vi "deliverWater_RIG1_cue.vi"() -> ()   [LabVIEW 2017]
uses:
  <vilib>/DAQmx/write.llb/DAQmx Write (Digital 1D Bool NChan 1Samp 1Line).vi
  <vilib>/DAQmx/create/channels.llb/DAQmx Create Channel (DO-Digital Output).vi
  <vilib>/DAQmx/miscellaneous.llb/DAQmx Fill In Error Info.vi
panel:
  in  "element":tag="Dev1/port0/line0"
  in  "Water on time (ms)":i32=100
  # "RIG 1"
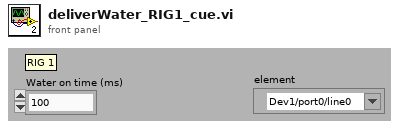
[diagram p1: front panel]
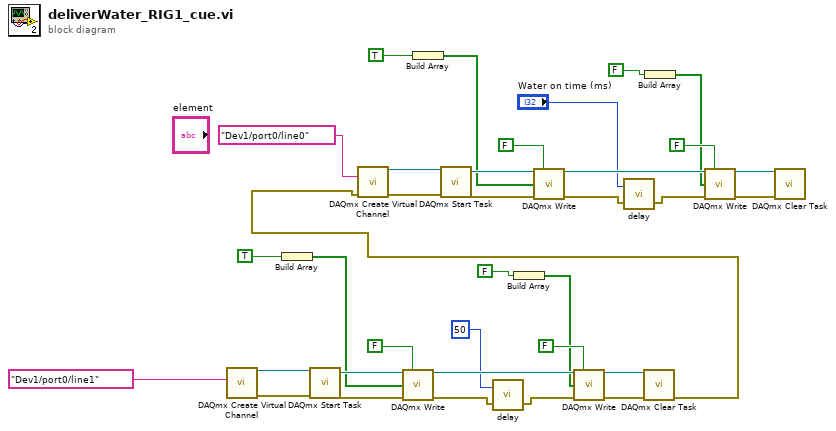
[diagram p0: block diagram]
diagram:
  n1 = call-poly <vilib>:"DAQmx Create Virtual Channel.vi"("lines"=tag "Dev1/port0/line1") -> ("task out"=w17:refnum<k21>, "error out"=w18:errorcluster)  [unwired: 6 in, 7 out]
  n2 = Build Array(TRUE ("auto start")) -> (w6:bool[])
  n3 = call <vilib>:"DAQmx Start Task.vi"("task/channels in"=w17, "error in"=w18) -> ("task out"=w16:refnum<k21>, "error out"=w15:errorcluster)  [unwired: 12 out]
  n4 = call-poly <vilib>:"DAQmx Write.vi"("task/channels in"=w16, "auto start"=FALSE, "data"=w6, "error in"=w15) -> ("task out"=w12:refnum<k21>, "error out"=w10:errorcluster)  [unwired: 10 out]
  n5 = Build Array(TRUE ("auto start")) -> (w21:bool[])
  n6 = call "delay.vi"("error in (no error)"=w10, "Delay (ms)"=u32 50) -> ("error out"=w11:errorcluster)  [unwired: 1 in]
  n7 = Build Array(FALSE ("auto start")) -> (w4:bool[])
  n8 = call-poly <vilib>:"DAQmx Write.vi"("task/channels in"=w12, "auto start"=FALSE, "data"=w4, "error in"=w11) -> ("task out"=w13:refnum<k21>, "error out"=w14:errorcluster)  [unwired: 10 out]
  n9 = call <vilib>:"DAQmx Clear Task.vi"("task in"=w13, "error in"=w14) -> ("error out"=w1:errorcluster)  [unwired: 13 out]
  n10 = call-poly <vilib>:"DAQmx Create Virtual Channel.vi"("lines"=tag "Dev1/port0/line0" ("element"), "error in"=w1) -> ("task out"=w33:refnum<k21>, "error out"=w35:errorcluster)  [unwired: 5 in, 7 out]
  n11 = call <vilib>:"DAQmx Start Task.vi"("task/channels in"=w33, "error in"=w35) -> ("task out"=w32:refnum<k21>, "error out"=w31:errorcluster)  [unwired: 12 out]
  n12 = call-poly <vilib>:"DAQmx Write.vi"("task/channels in"=w32, "auto start"=FALSE, "data"=w21, "error in"=w31) -> ("task out"=w28:refnum<k21>, "error out"=w25:errorcluster)  [unwired: 10 out]
  n13 = call "delay.vi"("error in (no error)"=w25, "Delay (ms)"="Water on time (ms)") -> ("error out"=w26:errorcluster)  [unwired: 1 in]
  n14 = Build Array(FALSE ("auto start")) -> (w19:bool[])
  n15 = call-poly <vilib>:"DAQmx Write.vi"("task/channels in"=w28, "auto start"=FALSE, "data"=w19, "error in"=w26) -> ("task out"=w29:refnum<k21>, "error out"=w30:errorcluster)  [unwired: 10 out]
  n16 = call <vilib>:"DAQmx Clear Task.vi"("task in"=w29, "error in"=w30) -> ()  [unwired: 14 out]
